vi "dummy F-70 controller.vi"() -> ()   [LabVIEW 2021, in "F-70 controller.lvlib"]
uses:
  F-70 controller.lvlib
  controls/F-70 controller states.ctl
  controls/F-70 controller commands.ctl
  controls/Message to F-70 controller.ctl
  controls/F-70 controller properties.ctl
panel:
  in  "Update interval (ms)":i32=5000
  in  "error in (no error)":errorcluster
  out "error out":errorcluster
  in  "F-70 contoller queue":refnum<queue>
  in  "Top queue":refnum<queue>
  in  "Start Stop btn":bool
  in  "Connect btn":bool
  in  "VISA resource name":refnum<visa-resource-name>
  # "Dummy F-70 controller"
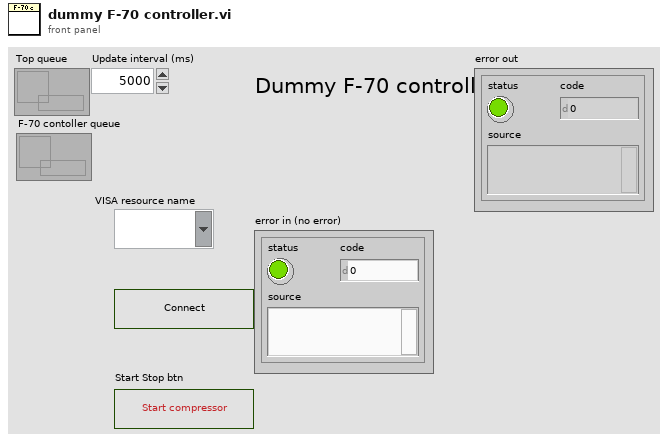
[diagram p1: front panel]
types:
  T1 = typedef "F-70 controller properties.ctl" = cluster{"Connected":bool, "Command msg":T2, "Data msg":variant, "Waiting msgs":i32, "Timeout counter":i32, "Logs":string[]}
  T2 = typedef "F-70 controller commands.ctl" = enum16{"Ignore", "Connect", "Read temperatures", "Read pressure", "Read status", "Update all", "Start compressor", "Stop compressor", "Clear error", "Disconnect"}
  T3 = typedef "F-70 controller.lvlib/F-70 controller states.ctl" = enum16{"Initialize GUI", "Wait for event", "Check message", "Execute command", "Send response", "Sleep", "Reserved", "Reserved2", "End"}
  T4 = typedef "Message to F-70 controller.ctl" = cluster{"Command msg":T2, "Data msg":variant}
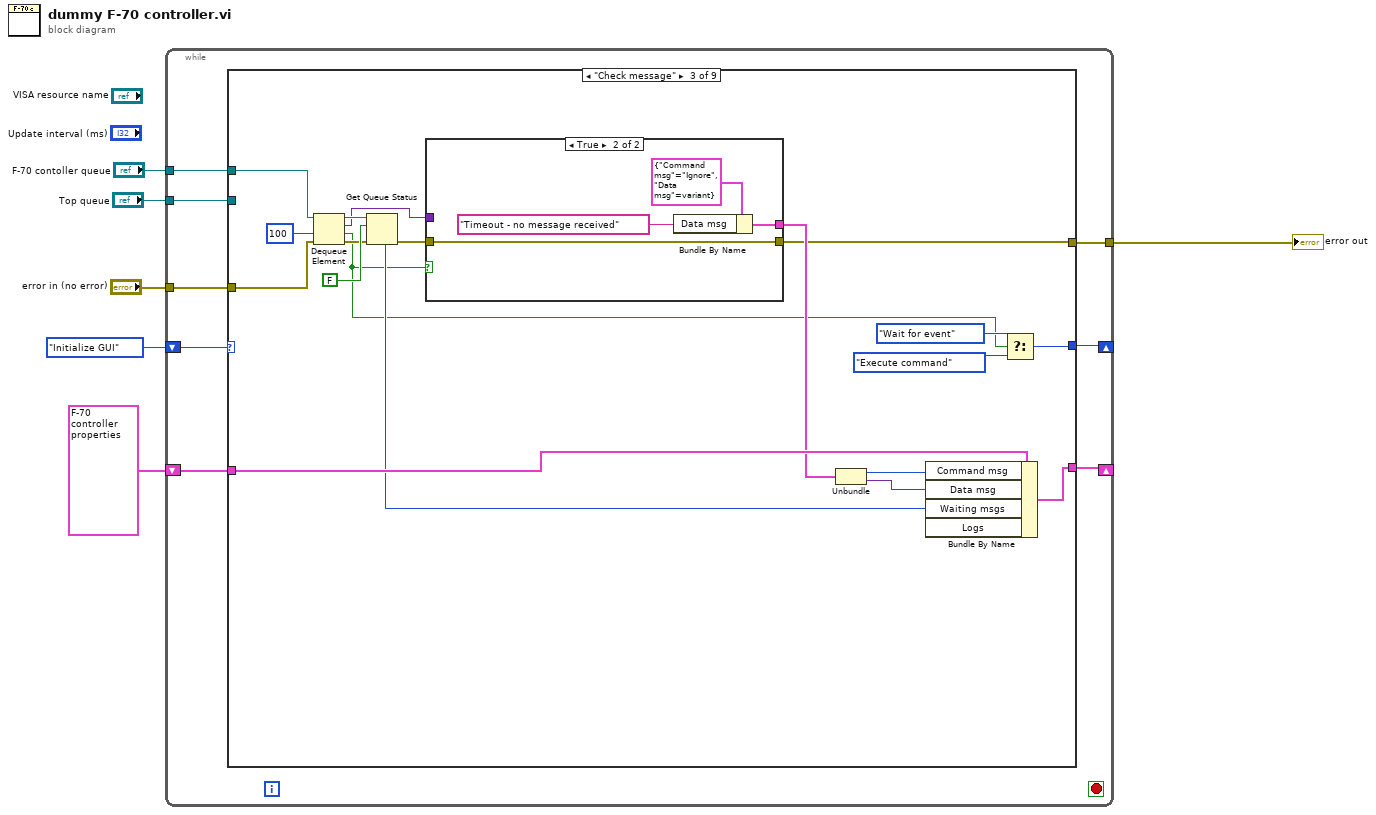
[diagram p0: block diagram]
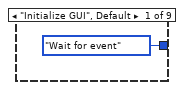
[diagram p2: hidden frame]
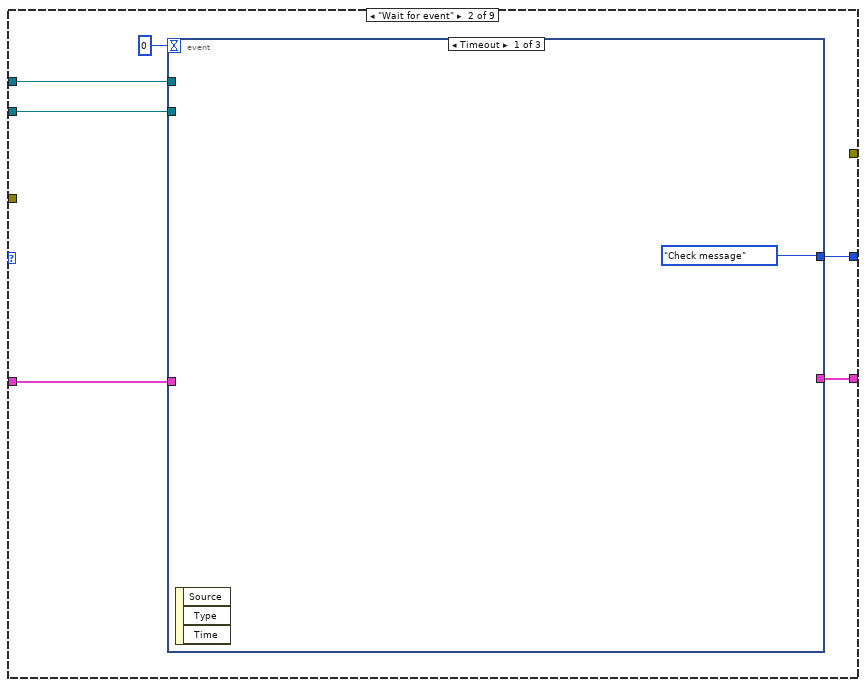
[diagram p3: hidden frame]
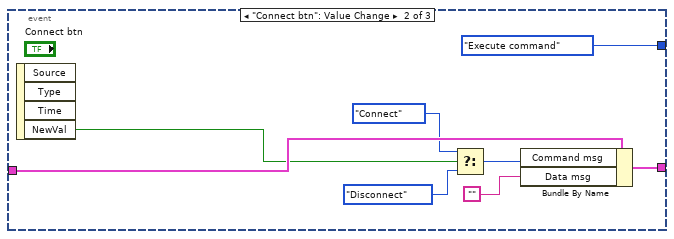
[diagram p4: hidden frame]
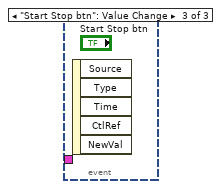
[diagram p5: hidden frame]
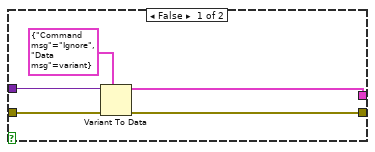
[diagram p6: hidden frame]
diagram:
  n1 = while {
    shift-right: [w13] -> _
    shift-left: F-70_controller_states."Initialize GUI" -> [w14]
    shift-right: [w11] -> _
    shift-left: T1 {"Connected"=FALSE, "Command msg"=enum."Ignore", "Data msg"=variant, "Waiting msgs"=0, "Timeout counter"=0, "Logs"=[]} ("F-70 controller properties") -> [w12]
    tunnel: "F-70 contoller queue" -> [w10]
    tunnel: "Top queue" -> [w9]
    tunnel: "error in (no error)" -> [w8]
    tunnel: [w7] -> w1
    stop <- _ stop-if-true
    n2 = case shown="\"Check message\"" w14 {
      tunnel: [F-70_controller_states."Wait for event" w20 w34 _ _ _ _ _ _] -> w13
      tunnel: w12 -> [_ w19 w43 _ _ _ _ _ _]
      tunnel: [_ w18 w37 _ _ _ _ _ _] -> w11
      tunnel: w10 -> [_ w17 w45 _ _ _ _ _ _]
      tunnel: w9 -> [_ w16 _ _ _ _ _ _ _]
      tunnel: w8 -> [_ _ w44 _ _ _ _ _ _]
      tunnel: [_ _ w35 _ _ _ _ _ _] -> w7
      frame "Initialize GUI", Default {
      }
      frame "Wait for event" {
        n3 = event shown="[0] Timeout" {
          selector: _ -> [_ _ _]
          dyn-events: _ -> [_ _ _]
          timeout: 0 -> [_ _ _]
          tunnel: [F-70_controller_states."Check message" F-70_controller_states."Execute command" _] -> w20
          tunnel: w19 -> [_ w28 _]
          tunnel: [_ w29 _] -> w18
          tunnel: w17 -> [_ _ _]
          tunnel: w16 -> [_ _ _]
          event Timeout {
            n4 = event-data() -> ()  [unwired: 1 in, 3 out]
          }
          event "Connect btn": Value Change {
            n5 = event-data() -> ("NewVal"=w24:bool)  [unwired: 1 in, 3 out]
            n6 = Select(t=F-70_controller_commands."Connect" ("Command msg"), s=w24, f=F-70_controller_commands."Disconnect") -> (s? t:f=w27:T2)
            n7 = Bundle By Name(cluster=w28, "Command msg"=w27, "Data msg"="") -> (w29:T1)
          }
          event "Start Stop btn": Value Change {
            n8 = event-data() -> ()  [unwired: 1 in, 5 out]
          }
        }
      }
      frame "Check message" {
        n9 = Dequeue Element(queue=w45, timeout in ms (-1)=100, error in (no error)=w44) -> (queue out=w46:refnum<queue>, element=w42:variant, timed out?=w32:bool, error out=w47:errorcluster)
        n10 = Get Queue Status(queue=w46, return elements? (F)=FALSE, error in (no error)=w47) -> (error out=w41:errorcluster, # elements in queue=w36:i32)  [unwired: 6 out]
        n11 = case shown="True" w32 {
          tunnel: w42 -> [w54 _]
          tunnel: w41 -> [w52 w58]
          tunnel: [w51 w56] -> w40
          tunnel: [w50 w58] -> w35
          frame False {
            n12 = Variant To Data(error in=w52, type=T4 {"Command msg"=enum."Ignore", "Data msg"=variant}, Variant=w54) -> (data=w51:T4, error out=w50:errorcluster)
          }
          frame True {
            n13 = Bundle By Name(cluster=T4 {"Command msg"=enum."Ignore", "Data msg"=variant}, "Data msg"="Timeout - no message received") -> (w56:T4)
          }
        }
        n14 = Unbundle(w40) -> ("Command msg"=w38:T2, "Data msg"=w39:variant)
        n15 = Bundle By Name(cluster=w43, "Command msg"=w38, "Data msg"=w39, "Waiting msgs"=w36) -> (w37:T1)  [unwired: 1 in]
        n16 = Select(t=F-70_controller_states."Wait for event", s=w32, f=F-70_controller_states."Execute command") -> (s? t:f=w34:T3)
      }
      frame "Execute command" {
      }
      frame "Send response" {
      }
      frame "Sleep" {
      }
      frame "Reserved" {
      }
      frame "Reserved2" {
      }
      frame "End" {
      }
    }
  }
  "error out" <- w1
